vi "Working Thread.vi"(8 "error in (no error)":errorcluster) -> (0 "error out":errorcluster)   [LabVIEW 2017, in "WebServiceImporter.lvlib" / "Main Panel.lvlib" / "Progress.lvlib"]
uses:
  <vilib>/Platform/WebService/Main Panel/Pages/Progress/Progress.lvlib
  <vilib>/Platform/WebService/Main Panel/Events/Data Type/Page.ctl
  <vilib>/Platform/WebService/Main Panel/Events/Events.lvlib
  <vilib>/Platform/WebService/ProxyDll Generator/ProxyDll Generator.lvlib
  <vilib>/Platform/WebService/VI Generator/VI Generator.lvlib
  <vilib>/Platform/WebService/Error Handling/Error Handling.lvlib
  <resource>/importtools/NISH Report/NISH Report.lvlib
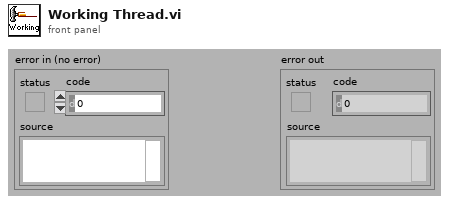
[diagram p1: front panel]
types:
  T1 = typedef "WebServiceImporter.lvlib/Main Panel.lvlib/Events.lvlib/Page.ctl" = enum16{"Input WSDL", "Input Authentication", "Input Info", "Select Methods", "Preview", "Progress", "Finish"}
  T2 = typedef "NISH Report.lvlib/Generate Report Object Reference.ctl" = refnum<k1>
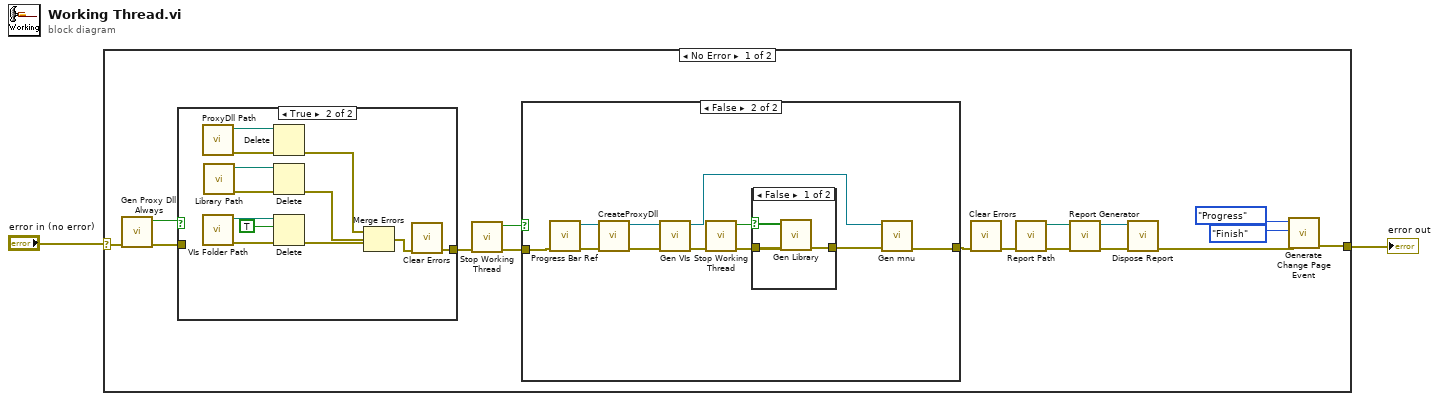
[diagram p0: block diagram]
diagram:
  n1 = case shown="No Error" "error in (no error)" {
    selector: "error in (no error)" -> [w10 w47]
    tunnel: [w15 w47] -> w1
    frame No Error {
      n2 = call <vilib>:"Gen Proxy Dll Always.vi"("error in (no error)"=w10) -> ("error out"=w8:errorcluster, "Generate whatever (out)"=w9:bool)  [unwired: 2 in, 7 out]
      n3 = case shown="True" w9 {
        tunnel: w8 -> [w19 _]
        tunnel: [w19 w24] -> w6
        frame False {
        }
        frame True {
          n4 = call <vilib>:"ProxyDll Path.vi"() -> ("error out"=w31:errorcluster, "ProxyDll Path (out)"=w30:path)  [unwired: 3 in, 7 out]
          n5 = call <vilib>:"VIs Folder Path.vi"() -> ("error out"=w27:errorcluster, "Path 2"=w26:path)  [unwired: 3 in, 7 out]
          n6 = call <vilib>:"Library Path.vi"() -> ("error out"=w29:errorcluster, "Path (out)"=w28:path)  [unwired: 3 in, 7 out]
          n7 = Delete(path (use dialog)=w30, error in=w31) -> (error out=w23:errorcluster)  [unwired: 5 out]
          n8 = Delete(path (use dialog)=w28, error in=w29) -> (error out=w22:errorcluster)  [unwired: 5 out]
          n9 = Delete(path (use dialog)=w26, entire hierarchy (F)=TRUE, error in=w27) -> (error out=w20:errorcluster)  [unwired: 4 out]
          n10 = Merge Errors(w23, w22, w20) -> (w21:errorcluster)
          n11 = call <vilib>:"Clear Errors.vi"("error in (no error)"=w21) -> ("error out"=w24:errorcluster)  [unwired: 1 in, 5 out]
        }
      }
      n12 = call <vilib>:"Stop Working Thread.vi"("error in (no error)"=w6) -> ("error out"=w7:errorcluster, "Stop the working thread(out)"=w18:bool)  [unwired: 2 in, 7 out]
      n13 = case shown="False" w18 {
        tunnel: [w32 w35] -> w14
        tunnel: w7 -> [w32 w37]
        frame True {
        }
        frame False {
          n14 = call <vilib>:"Progress Bar Ref.vi"("error in (no error)"=w37) -> ("error out"=w38:errorcluster, "Progress (out)"=w39:refnum<vi>)  [unwired: 2 in, 7 out]
          n15 = call <vilib>:"CreateProxyDll.vi"("error in (no error)"=w38, "Progress"=w39) -> ("error out"=w36:errorcluster, "Progress (out)"=w43:refnum<vi>)  [unwired: 8 out]
          n16 = call <vilib>:"Gen VIs.vi"("error in (no error)"=w36, "Progress"=w43) -> ("error out"=w42:errorcluster, "Progress (out)"=w33:refnum<vi>)  [unwired: 8 out]
          n17 = call <vilib>:"Stop Working Thread.vi"("error in (no error)"=w42) -> ("error out"=w40:errorcluster, "Stop the working thread(out)"=w41:bool)  [unwired: 2 in, 7 out]
          n18 = case shown="False" w41 {
            tunnel: w40 -> [w45 w46]
            tunnel: [w44 w46] -> w34
            frame False {
              n19 = call <vilib>:"Gen Library.vi"("error in (no error)"=w45) -> ("error out"=w44:errorcluster)  [unwired: 10 out]
            }
            frame True {
            }
          }
          n20 = call <vilib>:"Gen mnu.vi"("error in (no error)"=w34, "Progress"=w33) -> ("error out"=w35:errorcluster)  [unwired: 9 out]
        }
      }
      n21 = call <vilib>:"Clear Errors.vi"("error in (no error)"=w14) -> ("error out"=w13:errorcluster)  [unwired: 1 in, 5 out]
      n22 = call <vilib>:"Report Path.vi"("error in (no error)"=w13) -> ("error out"=w12:errorcluster, "Path (out)"=w11:path)  [unwired: 2 in, 7 out]
      n23 = call <vilib>:"Report Generator.vi"("error in (no error)"=w12, "Report File Path"=w11) -> ("error out"=w5:errorcluster, "report out"=w3:T2)  [unwired: 8 out]
      n24 = call <resource>:"Dispose Report.vi"("error in (no error)"=w5, "report in"=w3) -> ("error out"=w4:errorcluster)  [unwired: 5 out]
      n25 = call <vilib>:"Generate Change Page Event.vi"("error in (no error)"=w4, "Target Page"=Page."Finish", "Source Page"=Page."Progress") -> ("error out"=w15:errorcluster)  [unwired: 8 out]
    }
    frame Error {
    }
  }
  "error out" <- w1
